vi "SGUI Set Multiple Complex Values to Strings by Label.vi"(0 "labels (empty)":string, 1 "values (empty)":cdb[](array[numeric]), 2 "prefix (empty)":string, 3 "suffix (empty)":string, 5 "format string":string="%.6f", 7 "error in":errorcluster) -> (4 "assigned control refs":refnum<vi>[](array[refnum]), 8 "error out":errorcluster)   [LabVIEW 2020, in "varilib.lvlib"]
doc: "This VI formats complex values into 'pretty' strings and assigns it to into multiple string controls defined by control labels (must be registered first by calling 'SGUI Register Controls'). If multiple string control labels are assigned and just one number it will assign the number to all of them. If no value is assigned it will assign empty strings. It will generate error if control not found or has ivalid type but it ignores input errors (executes anyway)."
uses:
  varilib.lvlib
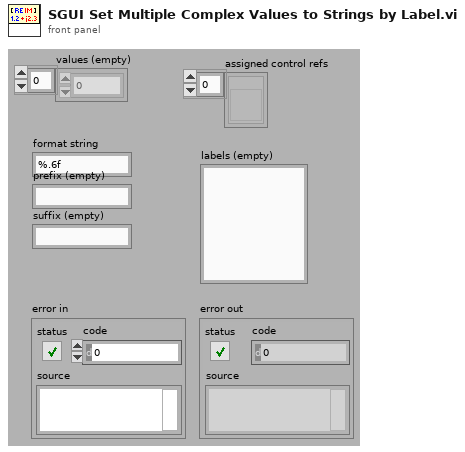
[diagram p1: front panel]
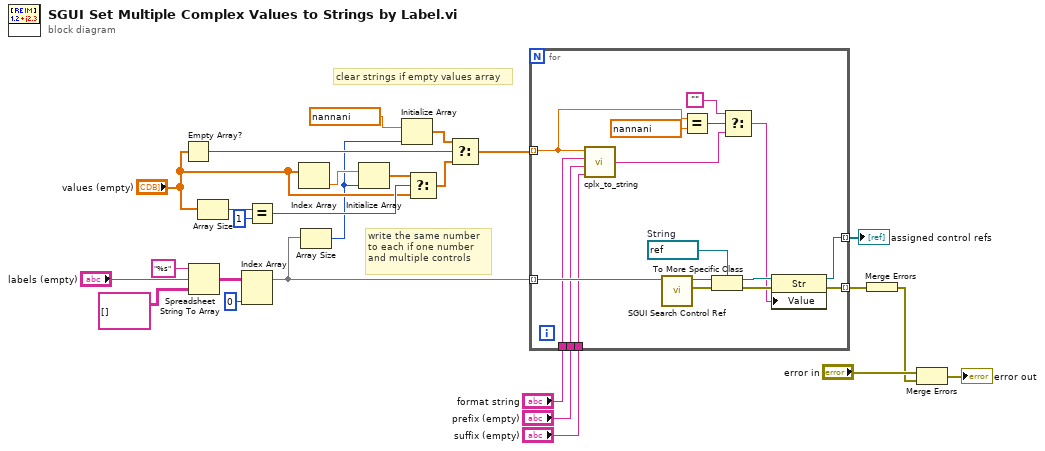
[diagram p0: block diagram]
diagram:
  # "write the same number\nto each if one number\nand multiple controls"
  # "clear strings if empty values array"
  n1 = Empty Array?(array="values (empty)") -> (empty?=w22:bool)
  n2 = Spreadsheet String To Array(format string="%s", spreadsheet string="labels (empty)", array type (2D Dbl)=string[][] []) -> (array=w23:string[][])  [unwired: 1 in]
  n3 = Array Size(array="values (empty)") -> (size(s)=w20:i32)
  n4 = Index Array(array=w23, index (col)=0 ("disabled index (col)")) -> (element=w11:string[])  [unwired: 1 in]
  n5 = Equal?(x=w20, y=1) -> (x = y?=w17:bool)
  n6 = Index Array(array="values (empty)") -> (element=w15:cdb)  [unwired: 1 in]
  n7 = Array Size(array=w11) -> (size(s)=w13:i32)
  n8 = Initialize Array(w15, w13) -> (w16:cdb[])
  n9 = Initialize Array(cdb nan+nani ("y"), w13) -> (w21:cdb[])
  n10 = Select(t=w16, s=w17, f="values (empty)") -> (s? t:f=w18:cdb[])
  n11 = Select(t=w21, s=w22, f=w18) -> (s? t:f=w12:cdb[])
  n12 = for {
    tunnel: w12 -> [w31] mode=indexing
    tunnel: w11 -> [w43] mode=indexing
    tunnel: [w33] -> w10 mode=indexing
    tunnel: [w32] -> w6 mode=indexing
    tunnel: "format string" -> [w29]
    tunnel: "prefix (empty)" -> [w28]
    tunnel: "suffix (empty)" -> [w27]
    w40 = refnum<vi> refnum  # String
    n13 = call "cplx_to_string.vi"("suffix (empty)"=w27, "prefix (empty)"=w28, "format string"=w29, "cplx in"=w31) -> ("formated string"=w30:string)
    n14 = call "SGUI Search Control Ref.vi"("control label (empty)"=w43) -> ("error out"=w42:errorcluster, "control ref out"=w41:refnum<vi>)  [unwired: 8 in, 1 out]
    n15 = Equal?(x=w31, y=cdb nan+nani) -> (x = y?=w37:bool)
    n16 = To More Specific Class(target class=w40, reference=w41, error in=w42) -> (specific class reference=w39:refnum<vi>, error out=w38:errorcluster)
    n17 = Select(t="", s=w37, f=w30) -> (s? t:f=w34:string)
    n18 = property class="Str"(reference=w39, error in=w38, "Value"=w34) -> (reference out=w32:refnum<vi>, error out=w33:errorcluster)
  }
  "assigned control refs" <- w6
  n19 = Merge Errors(w10) -> (w8:errorcluster)
  n20 = Merge Errors("error in", w8) -> (→"error out":errorcluster)
